vi "Init Username.vi"(8 "error in (no error)":errorcluster, 11 "[V] Login in":refnum<class "[V] Login.lvclass">) -> (0 "error out":errorcluster, 3 "[V] Login out":refnum<class "[V] Login.lvclass">)   [LabVIEW 2020, in "[V] Login.lvlib" / "[V] Login.lvclass"]
uses:
  [V] Login.lvclass
  [V] Login.lvclass/[V] Login.ctl
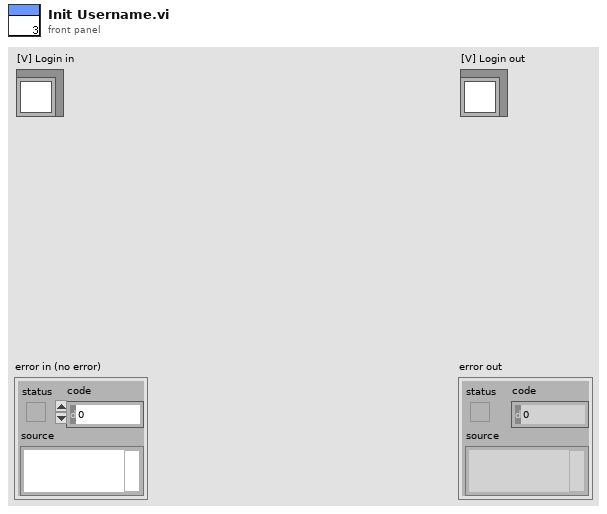
[diagram p1: front panel]
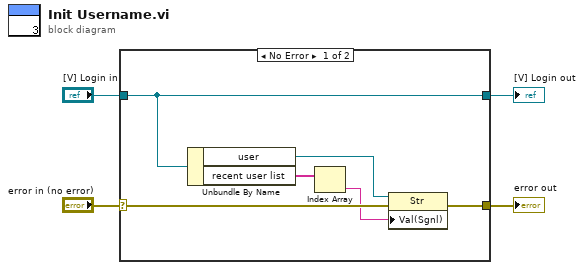
[diagram p0: block diagram]
diagram:
  n1 = case shown="No Error" "error in (no error)" {
    selector: "error in (no error)" -> [w9 w12]
    tunnel: [w5 w12] -> w3
    tunnel: [w10 w11] -> w1
    tunnel: "[V] Login in" -> [w10 w11]
    frame No Error {
      n2 = Unbundle By Name(w10) -> ("user"=w8:refnum<vi>, "recent user list"=w7:string[])
      n3 = Index Array(array=w7) -> (element=w6:string)  [unwired: 1 in]
      n4 = property class="Str"(reference=w8, error in=w9, "Val(Sgnl)"=w6) -> (error out=w5:errorcluster)  [unwired: 1 out]
    }
    frame Error {
    }
  }
  "error out" <- w3
  "[V] Login out" <- w1
